vi "Front End (1).vi"() -> ()   [LabVIEW 2015]
uses:
  <vilib>/Utility/file.llb/Write Delimited Spreadsheet (DBL).vi
panel:
  in  "Cluster":T1
  out "Cooler On":bool
  out "Heater on":bool
  out "Current Temperature":dbl
  out "?":dbl(slide) scale=0.0..35.0
  out "Temperature Over Time":cluster{i32[], dbl[]}(graph)
  in  "Temperature Scale":enum16{"Celsius", "Fahrenheit"}(ring)
  in  "stop":bool
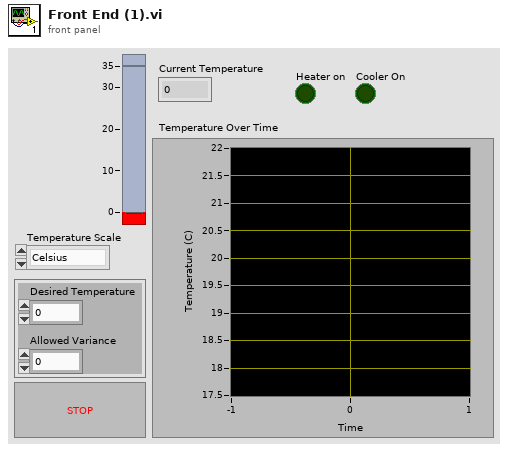
[diagram p1: front panel]
types:
  T1 = cluster{"Desired Temperature":dbl, "Allowed Variance":dbl}
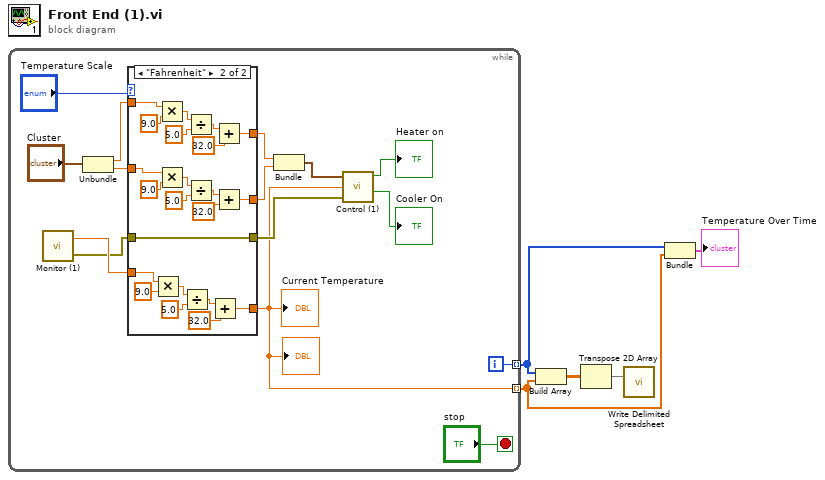
[diagram p0: block diagram]
diagram:
  n1 = while {
    tunnel: [w8] -> w2 mode=indexing
    tunnel: [w7] -> w3 mode=indexing
    i -> [w8]
    stop <- "stop" stop-if-true
    n2 = call "Monitor (1).vi"() -> ("error out"=w6:errorcluster, "data"=w19:dbl)
    n3 = Unbundle("Cluster") -> ("Desired Temperature"=w17:dbl, "Allowed Variance"=w16:dbl)
    n4 = case shown="\"Fahrenheit\"" "Temperature Scale" {
      tunnel: w19 -> [w22 w46]
      tunnel: [w22 w40] -> w7
      tunnel: w17 -> [w24 w30]
      tunnel: w16 -> [w23 w29]
      tunnel: [w23 w28] -> w14
      tunnel: [w24 w27] -> w15
      tunnel: w6 -> [w21 w25]
      tunnel: [w21 w25] -> w9
      frame "Celsius", Default {
      }
      frame "Fahrenheit" {
        n5 = Multiply(x=w46, y=9.0) -> (x*y=w44:dbl)
        n6 = Multiply(x=w30, y=9.0) -> (x*y=w39:dbl)
        n7 = Multiply(x=w29, y=9.0) -> (x*y=w34:dbl)
        n8 = Divide(x=w44, y=5.0) -> (x/y=w42:dbl)
        n9 = Divide(x=w39, y=5.0) -> (x/y=w37:dbl)
        n10 = Divide(x=w34, y=5.0) -> (x/y=w32:dbl)
        n11 = Add(x=w42, y=32.0) -> (x+y=w40:dbl)
        n12 = Add(x=w37, y=32.0) -> (x+y=w27:dbl)
        n13 = Add(x=w32, y=32.0) -> (x+y=w28:dbl)
      }
    }
    "?" <- w7
    "Current Temperature" <- w7
    n14 = Bundle("Desired Temperature"=w15, "Allowed Variance"=w14) -> (w13:T1)  [unwired: 1 in]
    n15 = call "Control (1).vi"("Cluster"=w13, "Current Temperature"=w7, "error in"=w9) -> ("Heater on"=→"Heater on":bool, "Cooler On"=→"Cooler On":bool)  [unwired: 2 out]
  }
  n16 = Build Array(w2, w3) -> (w5:dbl[][])
  n17 = Transpose 2D Array(2D array=w5) -> (transposed array=w4:dbl[][])
  n18 = call-poly <vilib>:"Write Delimited Spreadsheet.vi"("2D data"=w4) -> ()  [unwired: 13 in, 2 out]
  n19 = Bundle(w2, w3) -> (→"Temperature Over Time":cluster{i32[], dbl[]})  [unwired: 1 in]
